vi "PS_LCR_cal2.vi"(10 "Lower Voltge Limit":dbl=1.2, 11 "Upper Voltage Limit":dbl=4.0) -> (0 "Min":dbl, 1 "XY Graph":cluster{"Y":dbl[], "Y":dbl[]}[](graph)=[{"Y"=[0.0, 0.05, 0.1, 0.15, 0.2, 0.25, 0.3, 0.35, 0.4, 0.45, 0.5, 0.55, 0.6, 0.65, 0.7, 0.75, 0.8, 0.85, 0.9, 0.95, 1.0, 1.05, 1.1, 1.15, 1.2, 1.25, 1.3, 1.35, 1.4, 1.45, 1.5, 1.55, 1.6, 1.65, 1.7, 1.75, 1.8, 1.85, 1.9, 1.95, 2.0, 2.05, 2.1, 2.15, 2.2, 2.25, 2.3, 2.35, 2.4, 2.45, 2.5, 2.55, 2.6, 2.65, 2.7, 2.75, 2.8, 2.85, 2.9, 2.95, 3.0, 3.05, 3.1, 3.15, 3.2, 3.25, 3.3, 3.35, 3.4, 3.45, 3.5, 3.55, 3.6, 3.65, 3.7, 3.75, 3.8, 3.85, 3.9, 3.95, 4.0, 4.05, 4.1, 4.15, 4.2, 4.25, 4.3, 4.35, 4.4, 4.45, 4.5, 4.55, 4.6, 4.65, 4.7, 4.75, 4.8, 4.85, 4.9, 4.95, 5.0, 5.05], "Y"=[1.5298757135269085, 1.5328388976296985, 1.5293925856704482, 1.5345781578612852, 1.5339661959375244, 1.53018169447358, 1.5265743399104366, 1.5220007296691076, 1.51427068423586, 1.5063957004884947, 1.4997124321084379, 1.4819977450237825, 1.4447163815532993, 1.3573024588883174, 1.161603516393886, 0.820918029268634, 0.4199061821541399, 0.153622585843183, 0.15030511317271325, 0.43882866711630325, 0.9999006895515649, 1.7411958476019447, 2.5304981523045864, 3.255995414422078, 3.818694517751893, 4.165918458818913, 4.28151481082073, 4.198819455810404, 3.959059256056534, 3.6098544367966032, 3.1979556371752222, 2.7795023464614927, 2.353174058815591, 1.9588288800544416, 1.6140365864269837, 1.3070571708940657, 1.0370854125367381, 0.8146051627749571, 0.6324661084613775, 0.488896759796258, 0.3677123343585585, 0.27295498563700904, 0.2089245346149273, 0.1557966576810819, 0.11780676597356136, 0.09493875253211967, 0.08471256374939808, 0.07883451829497443, 0.07988129347656164, 0.08679000994821919, 0.1060506744395145, 0.11840262266212312, 0.14189870211324745, 0.16217393518736928, 0.18887475937212259, 0.21549506349261563, 0.24541673756696256, 0.27099026846865953, 0.29912437444837736, 0.32951307523590956, 0.3613189505652336, 0.3922229898377022, 0.4230787177962361, 0.44779873039006196, 0.4836145678075603, 0.509687339034607, 0.5342946249192798, 0.5705774896484697, 0.6011594528745015, 0.6259599926645998, 0.6571217110122272, 0.6779283991150254, 0.7090740151905816, 0.7342932688254709, 0.7632809176513753, 0.787839898681874, 0.815201020034375, 0.8366357778752933, 0.8612269695320995, 0.891003730987698, 0.9074461724203882, 0.9323916595874564, 0.957933004817351, 0.981493527508089, 1.0035080424099714, 1.0244435728298853, 1.046007169575612, 1.0641888732873335, 1.082000179455684, 1.1046749711119777, 1.124096703595656, 1.14831750481961, 1.1598159438564613, 1.180815894520082, 1.2004630880208707, 1.2108342296260255, 1.2341531943794966, 1.245104089613326, 1.2719659918665696, 1.2829813044791825, 1.3021775805287772, 1.3143201915840468]}], 2 "Min Voltage":dbl, 3 "Max Voltage":dbl)   [LabVIEW 2011]
uses:
  PS_Global.vi
  <vilib>/Instr/_visa.llb/VISA Configure Serial Port (Instr).vi
  <vilib>/Analysis/NI_AALBase.lvlib
panel:
  out "Max":dbl
  out "Waveform Chart 2":dbl(graph)
  in  "baud rate":u32=115200
  out "Waveform Chart":dbl(graph)
  out "Signal Mean":dbl format="%0.2f"
  out "Voltage 2 Setpoint":dbl
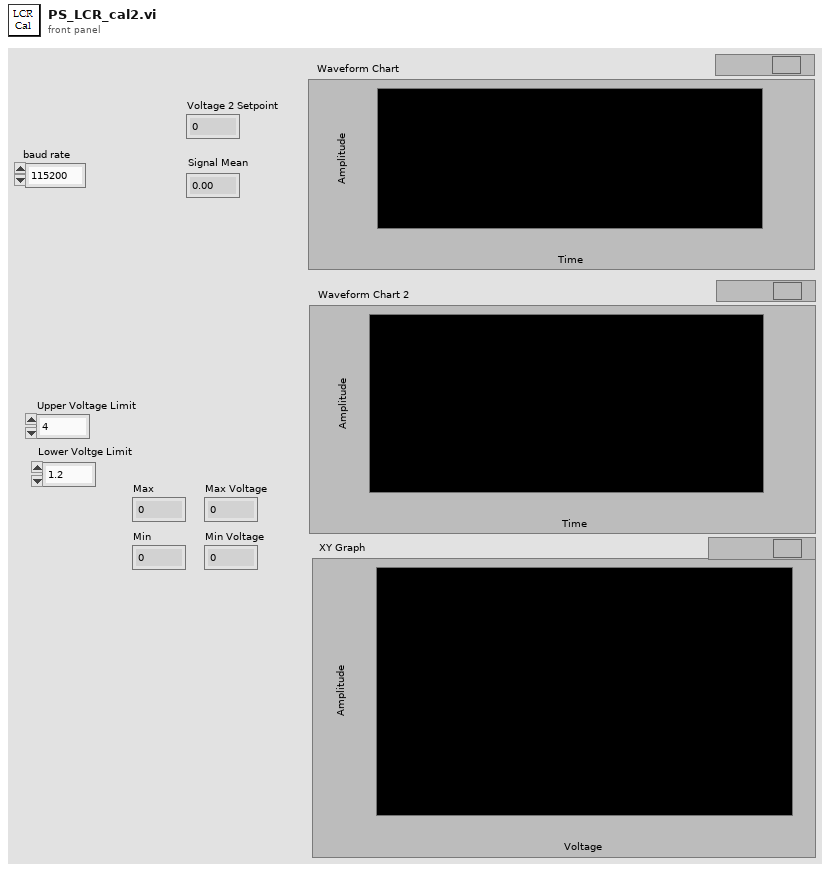
[diagram p1: front panel]
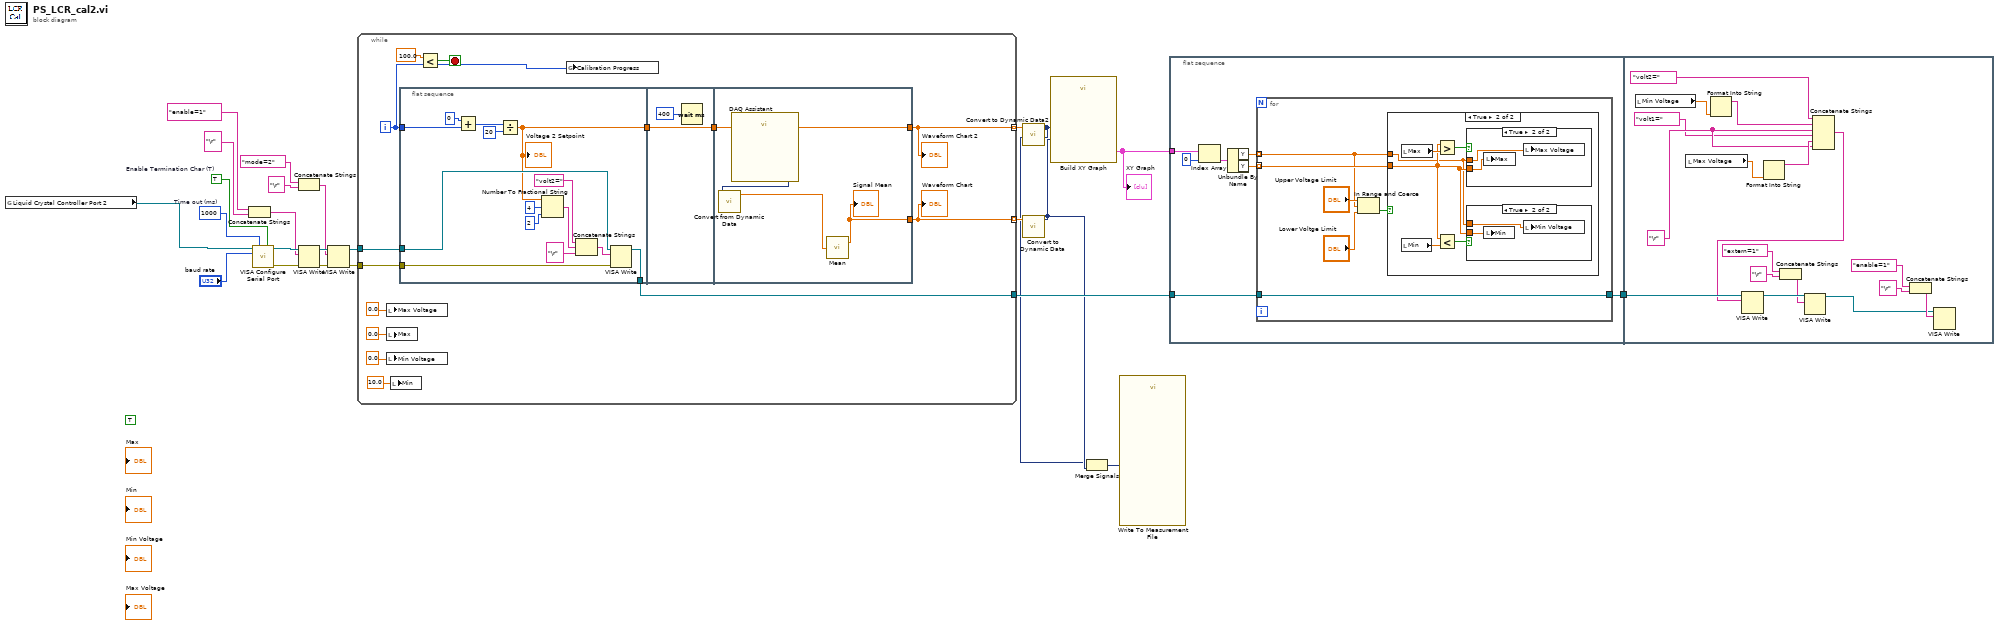
[diagram p0: block diagram]
diagram:
  (unwired) TRUE
  w20 = TRUE  # Enable Termination Char (T)
  w23 = 1000  # Time out (ms)
  n1 = global read "PS_Global.vi" "Liquid Crystal Controller Port 2"() -> (w1:refnum<visa-resource-name>)
  n2 = Concatenate Strings("enable=1", "\r") -> (w17:string)
  n3 = call-poly "VISA Configure Serial Port"("VISA resource name"=w1, "timeout (10sec)"=w23, "Enable Termination\nChar (T)"=w20, "baud rate (9600)"="baud rate") -> ("VISA resource name out"=w22:refnum<visa-resource-name>, "error out"=w21:errorcluster)  [unwired: 10 in]
  n4 = Concatenate Strings("mode=2" ("write buffer"), "\r") -> (w13:string)
  n5 = VISA Write(VISA resource name=w22, write buffer=w17, error in (no error)=w21) -> (VISA resource name out=w14:refnum<visa-resource-name>, error out=w12:errorcluster)  [unwired: 1 out]
  n6 = VISA Write(VISA resource name=w14, write buffer=w13, error in (no error)=w12) -> (VISA resource name out=w10:refnum<visa-resource-name>, error out=w11:errorcluster)  [unwired: 1 out]
  n7 = while {
    tunnel: w10 -> [w36]
    tunnel: w11 -> [w35]
    tunnel: [w32] -> w9 mode=indexing
    tunnel: [w31] -> w8 mode=indexing
    tunnel: [w26] -> w6
    i -> [w25]
    stop <- w37 stop-if-true
    n8 = local write "Max Voltage"(0.0 ("Max Voltage")) -> ()
    n9 = local write "Max"(0.0 ("Max")) -> ()
    n10 = local write "Min Voltage"(0.0 ("Min Voltage")) -> ()
    n11 = local write "Min"(10.0 ("Min")) -> ()
    n12 = flat-sequence {
      tunnel: w25 -> [w43]
      tunnel: w36 -> [w49]
      tunnel: w35 -> [w48]
      tunnel: [w40] -> w33
      tunnel: [w39] -> w26
      tunnel: [w53] -> w34
      tunnel: w33 -> [w53]
      tunnel: w34 -> [w56]
      tunnel: [w57] -> w32
      tunnel: [w56] -> w31
      frame #0 {
        n13 = Add(x=0, y=w43) -> (x+y=w44:i32)
        n14 = Divide(x=w44, y=20) -> (x/y=w40:dbl)
        "Voltage 2 Setpoint" <- w40
        n15 = Number To Fractional String(number=w40, width (-)=i16 4, precision (6)=i16 2) -> (F-format string=w47:string)  [unwired: 1 in]
        n16 = Concatenate Strings("volt2=" ("string"), w47, "\r") -> (w50:string)
        n17 = VISA Write(VISA resource name=w49, write buffer=w50, error in (no error)=w48) -> (VISA resource name out=w39:refnum<visa-resource-name>)  [unwired: 2 out]
      }
      frame #1 {
        n18 = Wait (ms)(milliseconds to wait=u32 400) -> ()  [unwired: 1 out]
      }
      frame #2 {
        n19 = call "DAQ Assistant"() -> ("data"=w58:dynamicdata)  [unwired: 17 in, 2 out]
        n20 = call "Convert from Dynamic Data"("Dynamic Data Type"=w58) -> ("Array"=w55:dbl[])  [unwired: 3 in]
        n21 = call <vilib>:"Mean.vi"("X"=w55) -> ("mean"=w57:dbl)  [unwired: 1 out]
        "Signal Mean" <- w57
      }
    }
    n22 = Less?(x=100.0, y=w25) -> (x < y?=w37:bool)
    n23 = global write "PS_Global.vi" "Calibration Progress"(w25) -> ()
    "Waveform Chart" <- w32
    "Waveform Chart 2" <- w31
  }
  n24 = call "Convert to Dynamic Data2"("Array"=w8) -> ("Dynamic Data Type"=w3:dynamicdata)  [unwired: 3 in]
  n25 = call "Convert to Dynamic Data"("Array"=w9) -> ("Dynamic Data Type"=w4:dynamicdata)  [unwired: 3 in]
  n26 = call "Build XY Graph"("Y Input"=w4, "X Input"=w3) -> ("XY Graph"=w7:cluster{"Y":dbl[], "Y":dbl[]}[])  [unwired: 3 in, 6 out]
  "XY Graph" <- w7
  n27 = Merge Signals(w3, w4) -> (w2:dynamicdata)
  n28 = call "Write To Measurement File"("Signals"=w2) -> ()  [unwired: 16 in, 3 out]
  n29 = flat-sequence {
    tunnel: w7 -> [w65]
    tunnel: w6 -> [w60]
    tunnel: [w59] -> w5
    tunnel: w5 -> [w98]
    frame #0 {
      n30 = Index Array(array=w65, index=0) -> (element=w63:cluster{"Y":dbl[], "Y":dbl[]})
      n31 = Unbundle By Name(w63) -> ("Y"=w62:dbl[], "Y"=w61:dbl[])
      n32 = for {
        tunnel: w62 -> [w67] mode=indexing
        tunnel: w61 -> [w68] mode=indexing
        tunnel: w60 -> [w66]
        tunnel: [w66] -> w59
        n33 = In Range and Coerce(upper limit="Upper Voltage Limit", x=w67, lower limit="Lower Voltge Limit") -> (In Range?=w71:bool)  [unwired: 1 out]
        n34 = case shown="True" w71 {
          tunnel: w68 -> [_ w73]
          tunnel: w67 -> [_ w72]
          frame False {
          }
          frame True {
            n35 = local read "Max"() -> (w75:dbl)
            n36 = local read "Min"() -> (w76:dbl)
            n37 = Greater?(x=w73, y=w75) -> (0:w74:bool)
            n38 = Less?(x=w73, y=w76) -> (x < y?=w77:bool)
            n39 = case shown="True" w74 {
              tunnel: w73 -> [_ w81]
              tunnel: w72 -> [_ w80]
              frame False {
              }
              frame True {
                n40 = local write "Max"(w81) -> ()
                n41 = local write "Max Voltage"(w80) -> ()
              }
            }
            n42 = case shown="True" w77 {
              tunnel: w73 -> [_ w79]
              tunnel: w72 -> [_ w78]
              frame False {
              }
              frame True {
                n43 = local write "Min"(w79) -> ()
                n44 = local write "Min Voltage"(w78) -> ()
              }
            }
          }
        }
      }
    }
    frame #1 {
      w91 = "\r"
      n45 = local read "Min Voltage"() -> (w96:dbl)
      n46 = local read "Max Voltage"() -> (w93:dbl)
      n47 = Format Into String(w96) -> (resulting string=w94:string)  [unwired: 3 in, 1 out]
      n48 = Format Into String(w93) -> (resulting string=w92:string)  [unwired: 3 in, 1 out]
      n49 = Concatenate Strings("extern=1" ("write buffer"), "\r") -> (w86:string)
      n50 = Concatenate Strings("volt2=" ("write buffer"), w94, w91, "volt1=" ("write buffer"), w92, w91) -> (w97:string)
      n51 = VISA Write(VISA resource name=w98, write buffer=w97) -> (VISA resource name out=w89:refnum<visa-resource-name>)  [unwired: 1 in, 2 out]
      n52 = VISA Write(VISA resource name=w89, write buffer=w86) -> (VISA resource name out=w82:refnum<visa-resource-name>)  [unwired: 1 in, 2 out]
      n53 = Concatenate Strings("enable=1" ("write buffer"), "\r") -> (w85:string)
      n54 = VISA Write(VISA resource name=w82, write buffer=w85) -> ()  [unwired: 1 in, 3 out]
    }
  }
